vi "Test Suite Result Published.vi"(8 "error in (no error)":errorcluster, 11 "Result Observation Test In":refnum<class "Result Observation Test.lvclass">) -> (0 "error out":errorcluster, 3 "Result Observation Test Out":refnum<class "Result Observation Test.lvclass">)   [LabVIEW 2020, in "Result Observation Test.lvclass"]
uses:
  Result Observation Test.lvclass
  Result Observation Test.lvclass/Result Observation Test.ctl
  Test Doubles/Test Case Test Double/Test Case Test Double.lvclass
  source/LUnit Test Suite.lvclass
  <vilib>/Astemes/LUnit/Test Case.lvclass
  source/Core/Result/Type.ctl
  source/Core/Result/Result.lvlib
  C:/git/astemes-lunit/source/Core/Runnable/Runnable.lvclass
  C:/Program Files (x86)/National Instruments/LabVIEW 2020/vi.lib/Astemes/LUnit/Test Case.lvclass
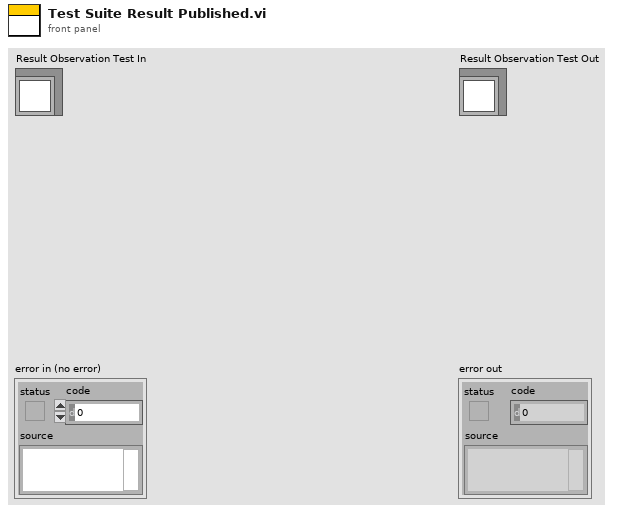
[diagram p1: front panel]
types:
  T1 = typedef "Result.lvlib/Result.ctl" = cluster{"Name":string, "Description":string, "Status":T2, "Result Type":T3, "Execution Time":dbl, "Data":cluster{"Expected":variant, "Actual":variant, "Delta":variant}}
  T2 = typedef "Result.lvlib/Status.ctl" = enum16{"", "Passed", "Failed", "Error", "Skipped", "Setup Error", "Broken", "Teardown Error"}
  T3 = typedef "Result.lvlib/Type.ctl" = enum16{"Test Case", "Test Suite", "Test Run", "Pass", "Fail", "Skip", "Pass if", "Fail if", "Pass if Error", "Fail if Error", "Pass if Equal", "Fail if Equal"}
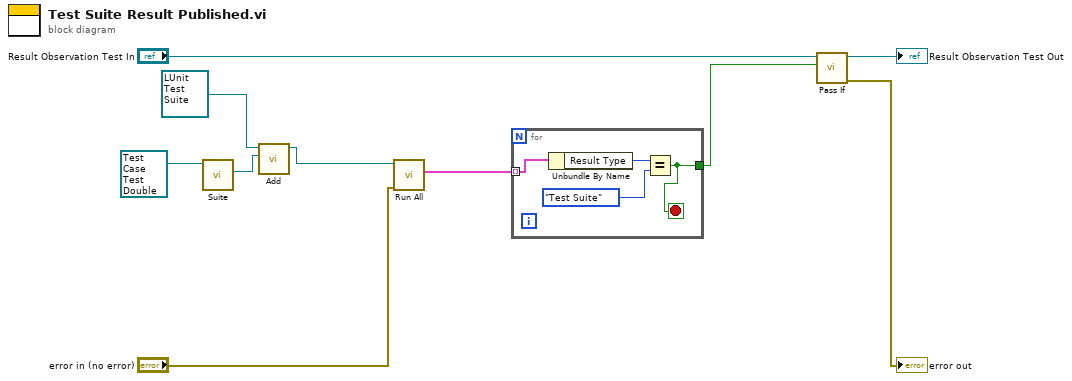
[diagram p0: block diagram]
diagram:
  n1 = call-dynamic "Suite.vi"("LUnit Test Case In"=refnum<class "Test Case Test Double.lvclass"> refnum ("LUnit Test Case V2 Test Double.lvclass")) -> ("LUnit Test Suite Out"=w1:refnum<class "LUnit Test Suite.lvclass">)  [unwired: 8 in, 2 out]
  n2 = call "Add.vi"("Runnable"=w1, "LUnit Test Suite In"=refnum<class "LUnit Test Suite.lvclass"> refnum ("LUnit Test Suite V2 in")) -> ("LUnit Test Suite Out"=w4:refnum<class "LUnit Test Suite.lvclass">)  [unwired: 8 in, 1 out]
  n3 = call "Run All.vi"("error in (no error)"="error in (no error)", "Runnable In"=w4) -> ("Results"=w3:T1[])  [unwired: 8 in, 1 out]
  n4 = for {
    tunnel: [w12] -> w2
    tunnel: w3 -> [w11] mode=indexing
    stop <- w12 stop-if-true
    n5 = Unbundle By Name(w11) -> ("Result Type"=w14:T3)
    n6 = Equal?(x=w14, y=Type."Test Suite" ("Result Type")) -> (x = y?=w12:bool)
  }
  n7 = call <vilib>:"Pass If.vi"("Pass?"=w2, "LUnit Test Case In"="Result Observation Test In") -> ("error out"=→"error out":errorcluster, "LUnit Test Case Out"=→"Result Observation Test Out":refnum<class "Result Observation Test.lvclass">)  [unwired: 8 in]
